vi "Obtain Request Events.vi"(8 "error in (no error)":errorcluster, 10 "Create New?":bool) -> (0 "error out":errorcluster, 2 "Actuator Module Request Events":T1)   [LabVIEW 2021, in "Actuator Module.lvlib"]
doc: "This VI Obtains/Creates the Requests events that will be used for other libraries to communicate with the library that owns this VI. These Requests events will be accessed only via Public API methods.\n\n<b>NOTE</b>: The contents of this VI are automatically generated and modified by the <b>Tools > Delacor > User Event</b> utilities. Consider using those utilities instead of making your own modifications to this VI.\n_______\nCreated using Delacor User Event Scripter 1.0.0.6."
uses:
  Actuator Module.lvlib
  Request Events--cluster.ctl
  Stop Argument--cluster.ctl
  Set Actuator Argument--cluster.ctl
panel:
  # "NOTE: The contents of this VI are automatically generated and modified by the Tools > Delacor > User Event utilities. Consider using those utilities instead of making your own modifications to this VI."
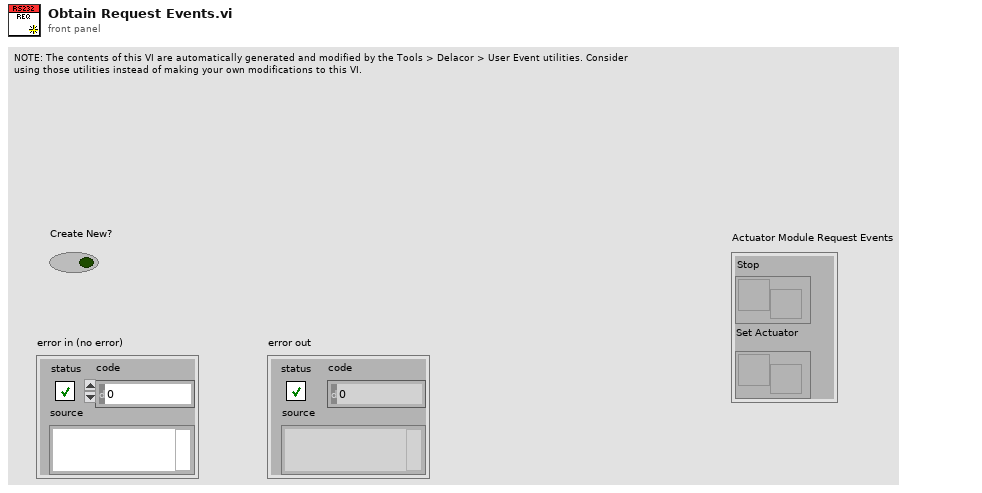
[diagram p1: front panel]
types:
  T1 = typedef "Actuator Module.lvlib/Request Events--cluster.ctl" = cluster{"Stop":refnum<user-event>, "Set Actuator":refnum<user-event>}
  T2 = typedef "Actuator Module.lvlib/Set Actuator Argument--cluster.ctl" = cluster{"Actuator":dbl}
  T3 = typedef "Actuator Module.lvlib/Stop Argument--cluster.ctl" = cluster{"Origin":string}
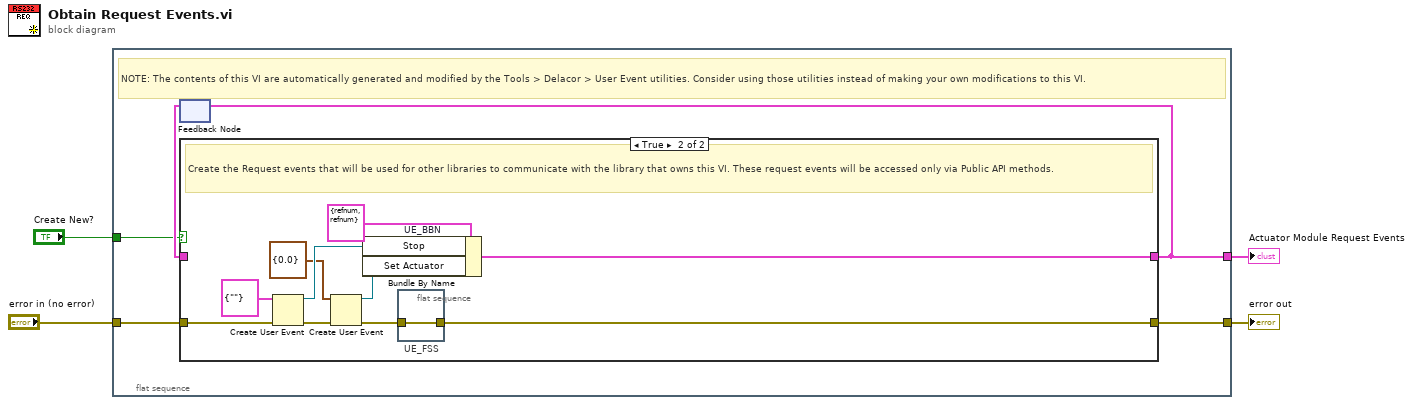
[diagram p0: block diagram]
diagram:
  n1 = flat-sequence {
    tunnel: [w9] -> w4
    tunnel: "error in (no error)" -> [w8]
    tunnel: [w6] -> w2
    tunnel: "Create New?" -> [w5]
    frame #0 {
      # "NOTE: The contents of this VI are automatically generated and modified by the Tools > Delacor > User Event utilities. Consider using those utilities instead of making your own modifications to this VI."
      n2 = feedback #1() -> (w7:T1)  [unwired: 1 in]
      n3 = case shown="True" w5 {
        tunnel: [w10 w15] -> w9
        tunnel: w8 -> [w10 w21]
        tunnel: [w11 w18] -> w6
        tunnel: w7 -> [w11 _]
        frame False {
          # "Obtain the Request events that were created in a previous call to this VI."
        }
        frame True {
          # "Create the Request events that will be used for other libraries to communicate with the library that owns this VI. These request events will be accessed only via Public API methods."
          n4 = Create User Event(user event datatype=T3 {"Origin"=""} ("Stop Argument"), error in=w21) -> (user event=w19:refnum<user-event>, error out=w16:errorcluster)
          n5 = Create User Event(user event datatype=T2 {"Actuator"=0.0} ("Set Actuator Argument"), error in=w16) -> (user event=w13:refnum<user-event>, error out=w14:errorcluster)
          n6 = Bundle By Name "UE_BBN"(cluster=T1 {"Stop"=refnum, "Set Actuator"=refnum} ("output cluster"), "Stop"=w19, "Set Actuator"=w13) -> (w18:T1)
          n7 = flat-sequence "UE_FSS" {
            tunnel: w14 -> [w22]
            tunnel: [w22] -> w15
            frame #0 {
            }
          }
        }
      }
      n8 = feedback-in #1(w6) -> ()
    }
  }
  "Actuator Module Request Events" <- w2
  "error out" <- w4
